vi "customController.vi"() -> ()   [LabVIEW 2020]
uses:
  <vilib>/Platform/TimedLoop/XDataNode/timing_clust.ctl
  <vilib>/Platform/TimedLoop/XDataNode/nitl_modes.ctl
  <vilib>/Platform/TimedLoop/XDataNode/wakeup.ctl
  <vilib>/rvi/Emulation/niFpgaSctlEmulationGetInTimedLoop.vi
  <vilib>/rvi/Emulation/niFpgaEmulationReportErrorSimple.vi
  <vilib>/rvi/Emulation/niFpgaGetClockAttributes.vi
  <vilib>/rvi/Emulation/niFpgaCriticalErrorInLSC.vi
  <vilib>/Platform/TimedLoop/XDataNode/XDataNode.xnode
  <vilib>/Platform/TimedLoop/XDataNode/XDNodeRunTimeDep.lvlib
panel:
  in  "max":fxp<+,15,-8>=0.00330197811126709 format="%#_51g"
  in  "min":fxp<+/-,15,-7>=-0.003301858901977539 format="%#_50g"
  in  "KiTs":fxp<+,11,-22>=1.25030055642128e-07 format="%#_61g"
  in  "Kp":fxp<+/-,32,-4>
  in  "TF Denominator":T1={"d2"=-5.379109252820069, "d3"=13.338745817780108, "d4"=-19.871028145479414, "d5"=19.50746353229121, "d6"=-13.043244632828106, "d7"=5.924549706009071, "d8"=-1.7592519447216297, "d9"=0.3093734613503629, "d10"=-0.024514322011746192} {"d10" format="%#_54g"; "d9" format="%#_52g"; "d8" format="%#_49g"; "d7" format="%#_49g"; "d6" format="%#_47g"; "d5" format="%#_47g"; "d4" format="%#_47g"; "d3" format="%#_47g"; "d2" format="%#_50g"}
  in  "TF Numerator":T2={"n2"=0.779209781450863, "n3"=-4.478196131314931, "n4"=12.236859326708696, "n5"=-20.5353561507535, "n6"=23.027520703445788, "n7"=-17.63415125244481, "n8"=9.00853418240981, "n9"=-2.8149211692703915, "n10"=0.41348492933818193} {"n10" format="%#_52g"; "n9" format="%#_51g"; "n8" format="%#_51g"; "n7" format="%#_51g"; "n6" format="%#_51g"; "n5" format="%#_51g"; "n4" format="%#_51g"; "n3" format="%#_51g"; "n2" format="%#_51g"}
  in  "Kp_Spool":fxp<+,10,14>=10000.0 format="%#_20g"
  in  "K_OL_RadSpool":fxp<+/-,10,-1>=0.14013671875 format="%#_64g"
  out "I_cmd":fxp<+/-,40,16>
  in  "xSpool_meas_m":fxp<+/-,32,-6>
  in  "ref_rad":fxp<+/-,32,-4>
  in  "reset":bool
  in  "meas_rad":fxp<+/-,32,-4>
  # "PI coefficients"
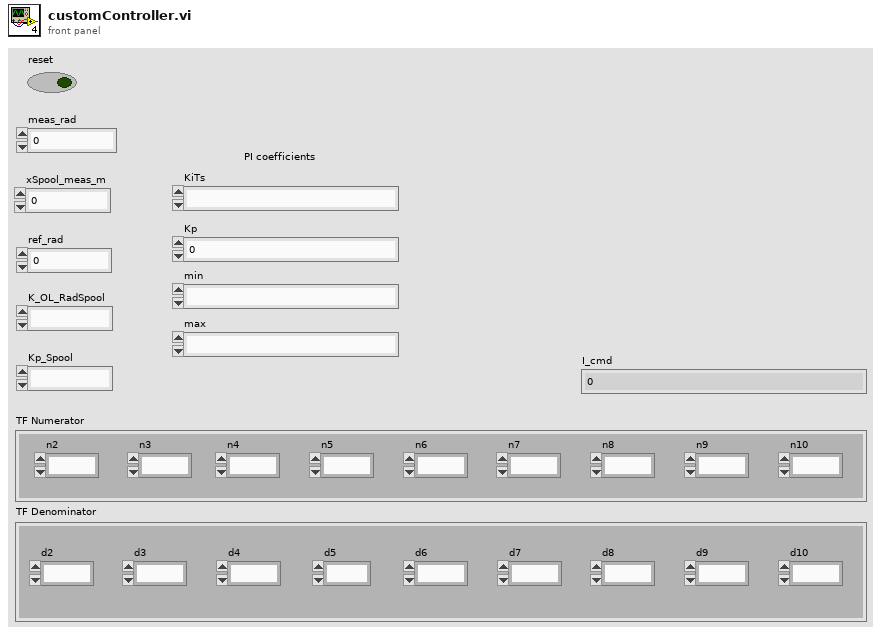
[diagram p1: front panel]
types:
  T1 = cluster{"d2":fxp<+/-,52,4>, "d3":fxp<+,49,4>, "d4":fxp<+/-,51,6>, "d5":fxp<+,50,5>, "d6":fxp<+/-,50,5>, "d7":fxp<+,51,3>, "d8":fxp<+/-,50,2>, "d9":fxp<+,51,-1>, "d10":fxp<+/-,51,-4>}
  T2 = cluster{"n2":fxp<+,51,0>, "n3":fxp<+/-,52,4>, "n4":fxp<+,49,4>, "n5":fxp<+/-,51,6>, "n6":fxp<+,50,5>, "n7":fxp<+/-,51,6>, "n8":fxp<+,52,4>, "n9":fxp<+/-,51,3>, "n10":fxp<+,51,-1>}
  T3 = typedef "XDNodeRunTimeDep.lvlib/timing_clust.ctl" = cluster{"Expected End [f-1]":u64, "Actual End [f-1]":u64, "Finished Late? [f-1]":bool, "Expected End [i-1]":u64, "Actual End [i-1]":u64, "Finished Late? [i-1]":bool, "Expected Start [i]":u64, "Actual Start [i]":u64, "Expected Start [f]":u64, "Actual Start [f]":u64, "Source Name":string, "Structure Name":string, "Period":i64, "Deadline":i64, "Offset":i64, "Start":i64, "Priority":i32, "Timeout":i32, "Mode":T4, "Wakeup Reason":T5, "Error":errorcluster, "Source Type":string, "Secondary Source Type":string, "Global End Time":u64, "Global Start Time":u64, "Frame Duration":u64, "Iteration Duration":u64, "Assigned CPU":i32, "I/O Scan Engine Mode":u32}
  T4 = typedef "XDNodeRunTimeDep.lvlib/nitl_modes.ctl" = enum32{"No Change", "Process missed periods, maintain original phase", "Discard missed periods, maintain original phase", "Process missed periods, ignore original phase", "Discard missed periods, ignore original phase"}
  T5 = typedef "XDNodeRunTimeDep.lvlib/wakeup.ctl" = enum32{"Normal", "Aborted", "Asynchronous wakeup", "Timing source error", "Timed loop error", "Timeout"}
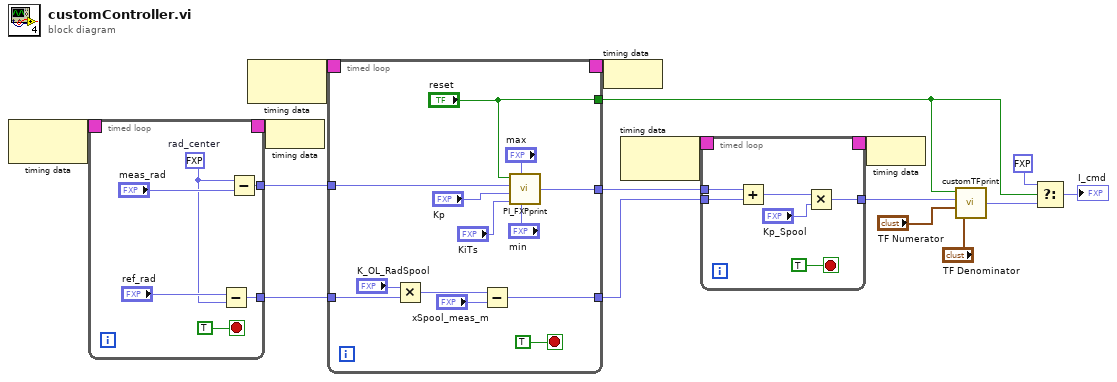
[diagram p0: block diagram]
diagram:
  n1 = node-c288() -> (w13:T3)  [unwired: 1 in]
  n2 = timed-loop {
    timing: w13 -> [_]
    timing-out: [_] -> w12
    tunnel: [w22] -> w7
    tunnel: [w18] -> w6
    stop <- TRUE stop-if-true
    w19 = fxp<+/-,1,1> 0.0  # rad_center
    n3 = Subtract(x="ref_rad", y=w19) -> (x-y=w18:fxp<+/-,32,-4>)
    n4 = Subtract(x=w19, y="meas_rad") -> (x-y=w22:fxp<+/-,32,-4>)
  }
  n5 = node-c288() -> (w17:T3)  [unwired: 1 in]
  n6 = node-c288(w12) -> ()
  n7 = timed-loop {
    timing: w17 -> [_]
    timing-out: [_] -> w16
    tunnel: [w34] -> w10
    tunnel: [w32] -> w11
    tunnel: ["reset"] -> w4
    tunnel: w7 -> [w30]
    tunnel: w6 -> [w33]
    stop <- TRUE stop-if-true
    n8 = Multiply(x="K_OL_RadSpool", y=w33) -> (x*y=w36:fxp<+/-,32,-7>)
    n9 = Subtract(x=w36, y="xSpool_meas_m") -> (x-y=w34:fxp<+/-,34,-6>)
    n10 = call "PI_FXPprint.vi"("min"="min", "max"="max", "KiTs"="KiTs", "Kp"="Kp", "e[k]"=w30, "reset"="reset") -> ("u[k]"=w32:fxp<+/-,47,-5>)
  }
  n11 = node-c288(w16) -> ()
  n12 = node-c288() -> (w15:T3)  [unwired: 1 in]
  n13 = timed-loop {
    timing: w15 -> [_]
    timing-out: [_] -> w14
    tunnel: w11 -> [w43]
    tunnel: w10 -> [w42]
    tunnel: [w41] -> w3
    stop <- TRUE stop-if-true
    n14 = Add(x=w43, y=w42) -> (x+y=w46:fxp<+/-,48,-4>)
    n15 = Multiply(x=w46, y="Kp_Spool") -> (x*y=w41:fxp<+/-,32,8>)
  }
  n16 = node-c288(w14) -> ()
  n17 = call "customTFprint.vi"("Denominator"="TF Denominator", "Numerator"="TF Numerator", "x[k]"=w3, "reset"=w4) -> ("y[k]"=w5:fxp<+/-,40,16>)
  n18 = Select(t=fxp<+/-,40,16> 0.0, s=w4, f=w5) -> (s? t:f=→"I_cmd":fxp<+/-,40,16>)
